vi "ma_Build BP & Estimate Order.vi"(3 "Desired Filter Specifications":T2 {"PB Gain" format="%0.2f"; "SB Gain" format="%0.2f"; "Lower SB" format="%0.2p"; "Upper SB" format="%0.2f"; "Lower PB" format="%0.2p"; "Upper PB" format="%0.2f"}, 4 "Filter type":T1(ring), 5 "Sampling Frequency":dbl format="%0.2f") -> (0 "filter order":i32=4 min=1 max=1000 step=1, 1 "Band Parameters":T3(array[cluster])=[{"amplitude"=0.0, "lower freq"=0.0, "higher freq"=0.13333333333333333, "ripple weight"=1.0}, {"amplitude"=1.001, "lower freq"=0.16666666666666666, "higher freq"=0.3, "ripple weight"=1.0}, {"amplitude"=0.0, "lower freq"=0.3333333333333333, "higher freq"=0.5, "ripple weight"=1.0}] {"amplitude" format="%0.4f"; "lower freq" format="%0.4f"; "higher freq" format="%0.4f"; "ripple weight" format="%0.4f"})   [LabVIEW 2020, in "NI_MAPro.lvlib"]
uses:
  NI_MAPro.lvlib
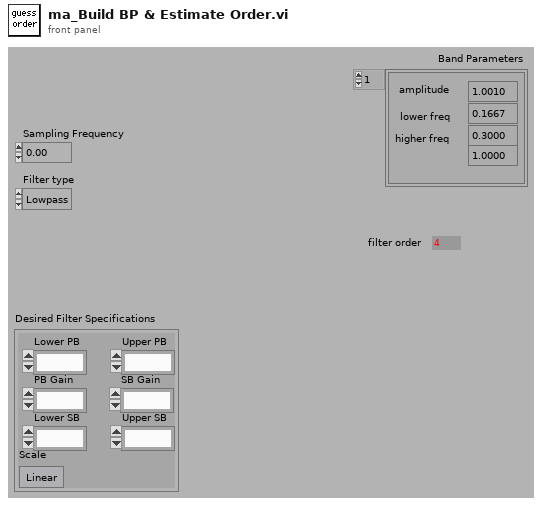
[diagram p1: front panel]
types:
  T1 = enum32{"Lowpass", "Highpass", "Bandpass", "Bandstop"}
  T2 = cluster{"Lower PB":dbl, "Upper PB":dbl, "Lower SB":dbl, "Upper SB":dbl, "PB Gain":dbl, "SB Gain":dbl, "Scale":bool}
  T3 = cluster{"amplitude":dbl, "lower freq":dbl, "higher freq":dbl, "ripple weight":dbl}[]
  T4 = enum32{"lowpass", "Highpass", "bandpass", "bandstop"}
  T5 = enum32{"lowpass", "highpass", "bandpass", "Bandstop"}
  T6 = cluster{dbl, "Lower SB":dbl, "Lower PB":dbl, dbl}[]
  T7 = cluster{dbl, "Lower PB":dbl, "Lower SB":dbl, dbl}[]
  T8 = cluster{dbl, "Lower PB":dbl, "Upper PB":dbl, dbl}
  T9 = cluster{dbl, "Upper SB":dbl, "Upper PB":dbl, dbl}[]
  T10 = cluster{dbl, "Lower SB":dbl, "Upper SB":dbl, dbl}
  T11 = cluster{dbl, "Upper PB":dbl, "Upper SB":dbl, dbl}[]
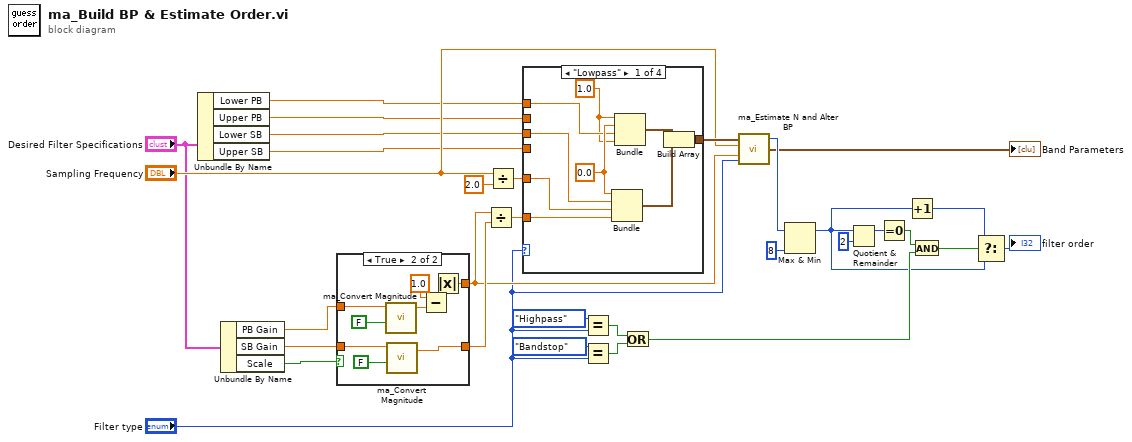
[diagram p0: block diagram]
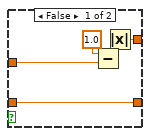
[diagram p2: hidden frame]
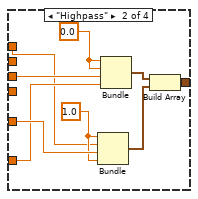
[diagram p3: hidden frame]
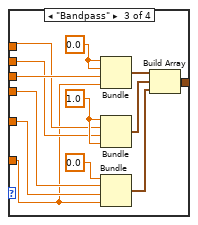
[diagram p4: hidden frame]
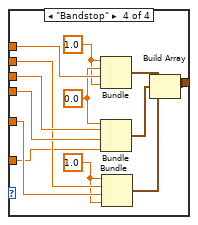
[diagram p5: hidden frame]
diagram:
  n1 = Unbundle By Name("Desired Filter Specifications") -> ("Lower PB"=w5:dbl, "Upper PB"=w6:dbl, "Lower SB"=w7:dbl, "Upper SB"=w8:dbl)
  n2 = Unbundle By Name("Desired Filter Specifications") -> ("PB Gain"=w1:dbl, "SB Gain"=w2:dbl, "Scale"=w3:bool)
  n3 = case shown="True" w3 {
    tunnel: [w33 w39] -> w31
    tunnel: [w34 w43] -> w27
    tunnel: w2 -> [w33 w37]
    tunnel: w1 -> [w32 w38]
    frame False {
      n4 = Subtract(x=1.0, y=w32) -> (x-y=w35:dbl)
      n5 = Absolute Value(x=w35) -> (abs(x)=w34:dbl)
    }
    frame True {
      n6 = call "ma_Convert Magnitude.vi"("conversion"=FALSE, "G in"=w38) -> ("G out"=w41:dbl)  [unwired: 2 in, 1 out]
      n7 = call "ma_Convert Magnitude.vi"("conversion"=FALSE, "G in"=w37) -> ("G out"=w39:dbl)  [unwired: 2 in, 1 out]
      n8 = Subtract(x=1.0, y=w41) -> (x-y=w44:dbl)
      n9 = Absolute Value(x=w44) -> (abs(x)=w43:dbl)
    }
  }
  n10 = Divide(x=w27, y=w31) -> (x/y=w30:dbl)
  n11 = Divide(x="Sampling Frequency", y=2.0) -> (x/y=w28:dbl)
  n12 = case shown="\"Lowpass\"" "Filter type" {
    tunnel: [w52 w61 w74 w88] -> w12
    tunnel: w5 -> [w51 w55 w70 w84]
    tunnel: w7 -> [w50 w56 w71 w83]
    tunnel: w30 -> [w48 w58 w64 w79]
    tunnel: w28 -> [w47 w60 w66 w86]
    tunnel: w6 -> [_ _ w69 w81]
    tunnel: w8 -> [_ _ w67 w82]
    frame "Lowpass" {
      w53 = 0.0
      w49 = 1.0
      n13 = Bundle(w53, "Lower SB"=w50, w47, w48) -> (w46:cluster{dbl, "Lower SB":dbl, dbl, dbl})  [unwired: 1 in]
      n14 = Bundle(w49, w53, "Lower PB"=w51, w49) -> (w54:cluster{dbl, dbl, "Lower PB":dbl, dbl})  [unwired: 1 in]
      n15 = Build Array(w54, w46) -> (w52:T6)
    }
    frame "Highpass" {
      w57 = 1.0
      w62 = 0.0
      n16 = Bundle(w57, "Lower PB"=w55, w60, w57) -> (w59:cluster{dbl, "Lower PB":dbl, dbl, dbl})  [unwired: 1 in]
      n17 = Bundle(w62, w62, "Lower SB"=w56, w58) -> (w63:cluster{dbl, dbl, "Lower SB":dbl, dbl})  [unwired: 1 in]
      n18 = Build Array(w63, w59) -> (w61:T7)
    }
    frame "Bandpass" {
      w72 = 1.0
      w75 = 0.0
      n19 = Bundle(w75, w75, "Lower SB"=w71, w64) -> (w76:cluster{dbl, dbl, "Lower SB":dbl, dbl})  [unwired: 1 in]
      n20 = Bundle(w72, "Lower PB"=w70, "Upper PB"=w69, w72) -> (w73:T8)  [unwired: 1 in]
      n21 = Bundle(0.0, "Upper SB"=w67, w66, w64) -> (w65:cluster{dbl, "Upper SB":dbl, dbl, dbl})  [unwired: 1 in]
      n22 = Build Array(w76, w73, w65) -> (w74:T9)
    }
    frame "Bandstop" {
      w78 = 1.0
      w80 = 0.0
      w77 = 1.0
      n23 = Bundle(w77, w80, "Lower PB"=w84, w77) -> (w89:cluster{dbl, dbl, "Lower PB":dbl, dbl})  [unwired: 1 in]
      n24 = Bundle(w80, "Lower SB"=w83, "Upper SB"=w82, w79) -> (w87:T10)  [unwired: 1 in]
      n25 = Bundle(w78, "Upper PB"=w81, w86, w78) -> (w85:cluster{dbl, "Upper PB":dbl, dbl, dbl})  [unwired: 1 in]
      n26 = Build Array(w89, w87, w85) -> (w88:T11)
    }
  }
  n27 = Equal?(x=T4."Highpass", y="Filter type") -> (x = y?=w24:bool)
  n28 = Equal?(x=T5."Bandstop", y="Filter type") -> (x = y?=w23:bool)
  n29 = Or(x=w24, y=w23) -> (x .or. y?=w19:bool)
  n30 = call "ma_Estimate N and Alter BP.vi"("type"="Filter type", "nominal ripple"=w27, "sampling freq"="Sampling Frequency", "Band Parameters In"=w12) -> ("Band Parameters Out"=→"Band Parameters":T3, "order"=w15:i32)  [unwired: 1 in]
  n31 = Max & Min(x=w15, y=8) -> (max(x,y)=w14:i32)  [unwired: 1 out]
  n32 = Quotient & Remainder(x=w14, y=2) -> (x-y*floor(x/y)=w21:i32)  [unwired: 1 out]
  n33 = Equal To 0?(x=w21) -> (x = 0?=w20:bool)
  n34 = Increment(x=w14) -> (x+1=w17:i32)
  n35 = And(x=w20, y=w19) -> (x .and. y?=w18:bool)
  n36 = Select(t=w17, s=w18, f=w14) -> (s? t:f=→"filter order":i32)
